vi "PFI-28000-28144-Demo_Main.vi"() -> ()   [LabVIEW 2017]
uses:
  PFI-28000-28144-Demo-State.ctl
  PFI-28000-28144-Demo-State Data.ctl
  28144 Card/PFI-28000-Card-28144.lvclass
  C:/wc/07143 Precision Filters 28000 Support/Driver/source/Card/PFI-28000-Card.lvclass
  28144 Channel/PFI-28000-Chan-28144.lvclass
  C:/wc/07143 Precision Filters 28000 Support/Driver/source/Bridge Channel/PFI-28000-Chan-Bridge.lvclass
  Card/PFI-28000-Card.lvclass
  Channel/PFI-28000-Channel.lvclass
  System/PFI-28000-System.lvclass
panel:
  in  "Type":enum16{"Low Pass Only", "Band Pass"}(ring)
  out "Auto Bal Status":string[](array[string])
  in  "Stop":bool
  in  "Auto Balance":bool[](array[boolean])
  out "Loop Resistance":dbl[](array[numeric])
  out "Excitation Current":dbl[](array[numeric])
  out "Identity":string
  out "Hostname":string
  in  "Gain":dbl[](array[numeric])
  in  "LP Filter Cutoff":dbl[](array[numeric])
  in  "Port":u16=28000
  in  "Address":string="169.254.1.221"
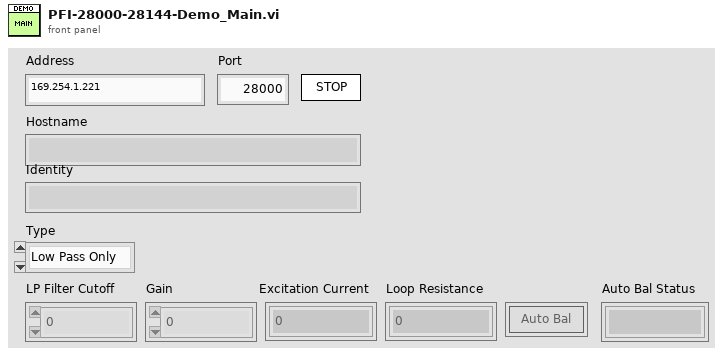
[diagram p1: front panel]
types:
  T1 = typedef "PFI-28000-28144-Demo-State Data.ctl" = cluster{"Card":refnum<class "PFI-28000-Card-28144.lvclass">, "Channels":refnum<class "PFI-28000-Chan-28144.lvclass">[]}
  T2 = typedef "PFI-28000-28144-Demo-State.ctl" = enum16{"InitDevice", "InitGUI", "HandleEvent"}
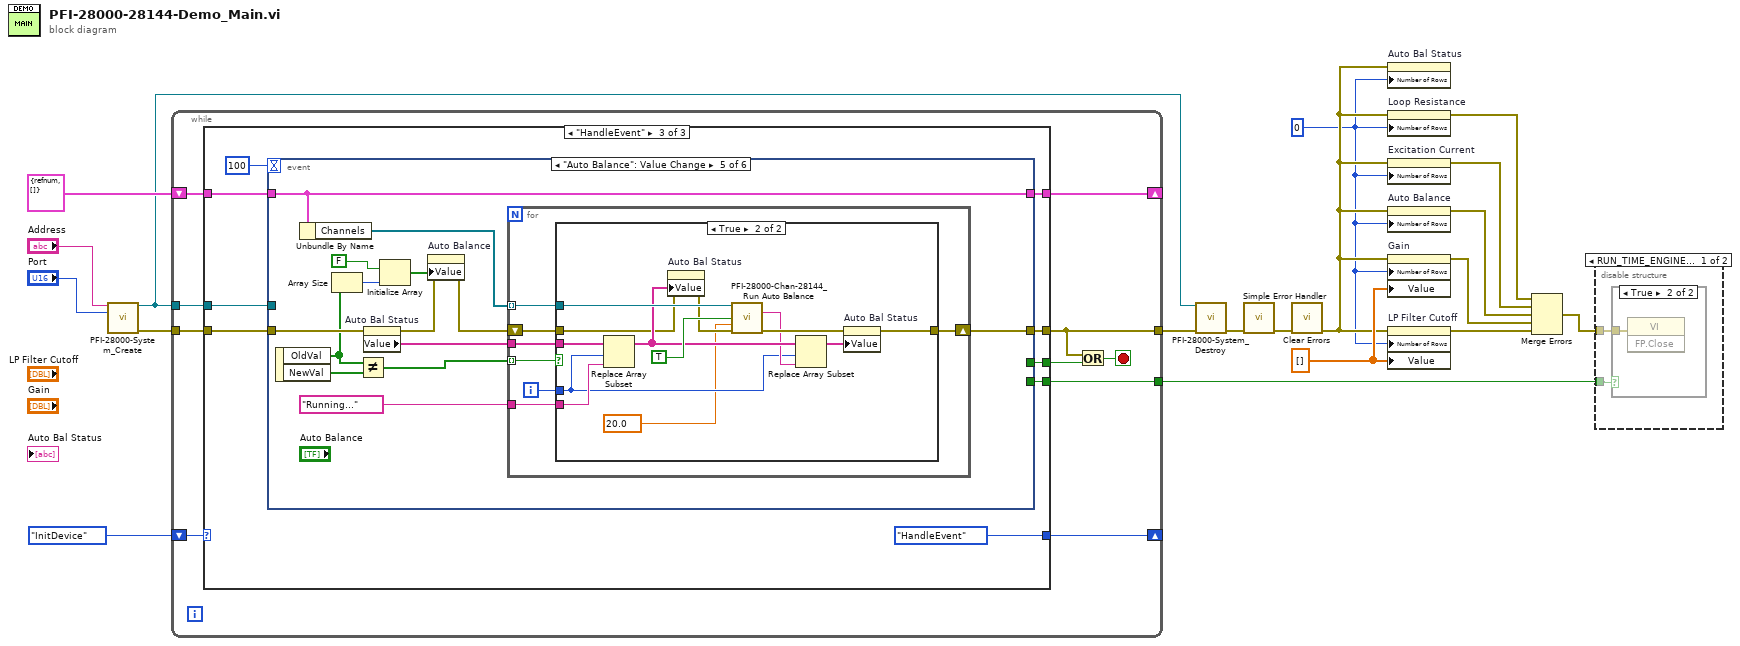
[diagram p0: block diagram]
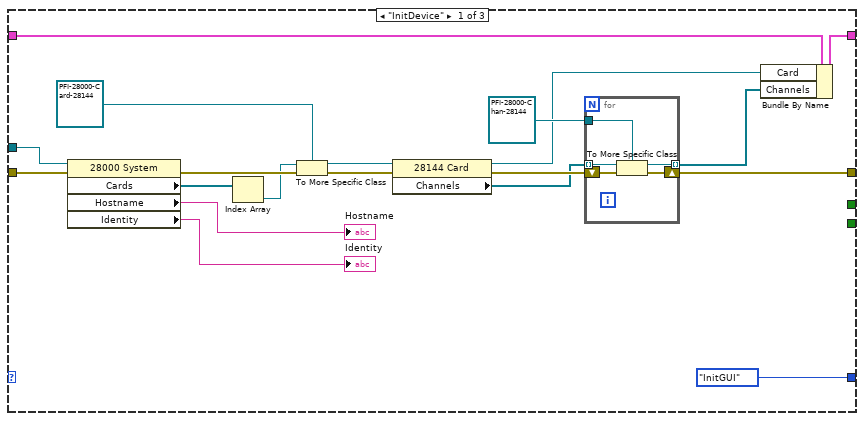
[diagram p4: hidden frame]
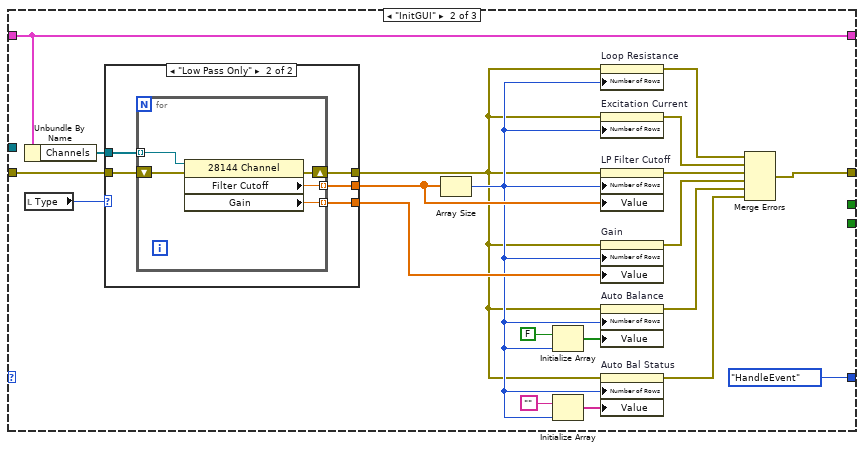
[diagram p5: hidden frame]
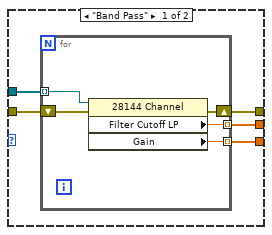
[diagram p6: hidden frame]
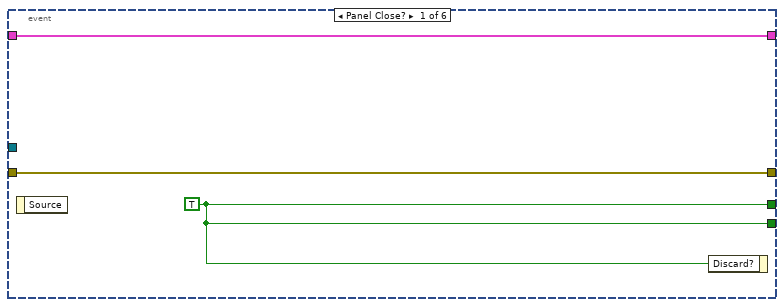
[diagram p7: hidden frame]
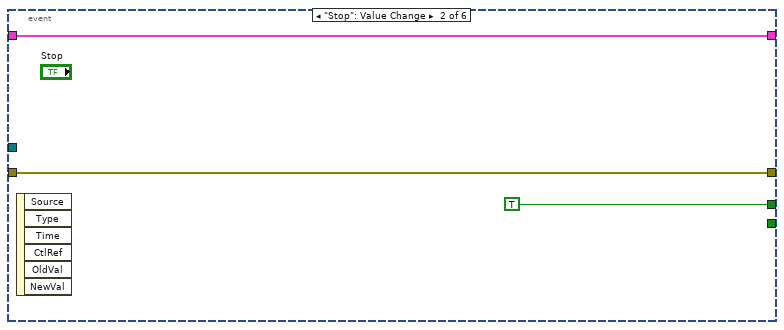
[diagram p8: hidden frame]
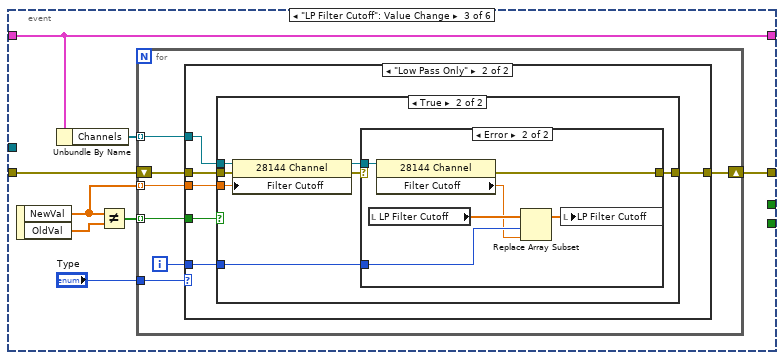
[diagram p9: hidden frame]
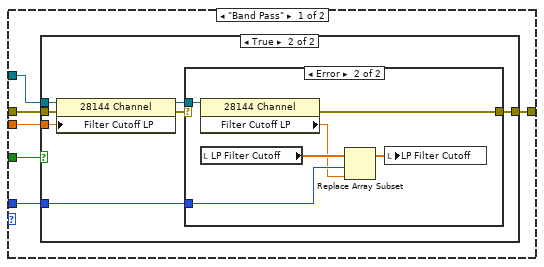
[diagram p10: hidden frame]
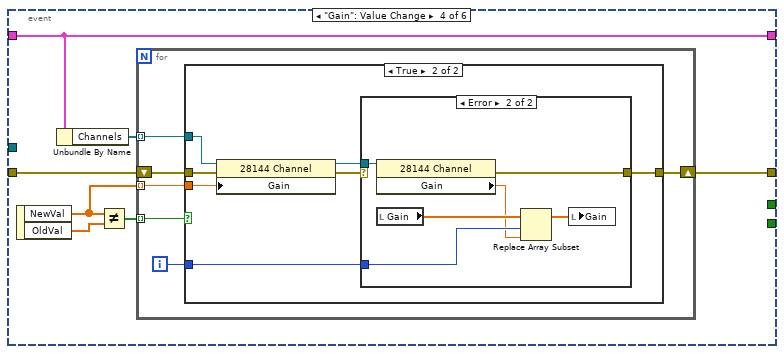
[diagram p15: hidden frame]
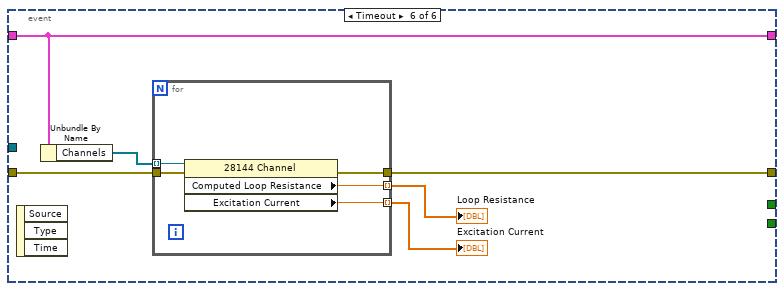
[diagram p19: hidden frame]
diagram:
  w10 = dbl[] [] ("Filter Cutoff")
  w2 = u32 0 ("Number of Rows")
  n1 = call "PFI-28000-System_Create.vi"("Address"="Address", "Port"="Port") -> ("PFI-28000-System out"=w13:refnum<class "PFI-28000-System.lvclass">, "error out"=w17:errorcluster)  [unwired: 12 in]
  n2 = while {
    tunnel: w17 -> [w29]
    tunnel: w13 -> [w27]
    shift-right: [w26] -> _
    shift-left: PFI-28000-28144-Demo-State."InitDevice" -> [w28]
    shift-right: [w24] -> _
    shift-left: T1 {"Card"=refnum, "Channels"=[]} ("Data") -> [w25]
    tunnel: [w23] -> w14
    tunnel: [w20] -> w1
    stop <- w22 stop-if-true
    n3 = case shown="\"HandleEvent\"" w28 {
      tunnel: w27 -> [w48 _ w102]
      tunnel: w29 -> [w47 w72 w101]
      tunnel: [PFI-28000-28144-Demo-State."InitGUI" PFI-28000-28144-Demo-State."HandleEvent" PFI-28000-28144-Demo-State."HandleEvent"] -> w26
      tunnel: [w37 w62 w98] -> w23
      tunnel: w25 -> [w36 w73 w97]
      tunnel: [w35 w73 w96] -> w24
      tunnel: [_ _ w99] -> w21
      tunnel: [_ _ w94] -> w20
      frame "InitDevice" {
        n4 = property class="28000 System"(reference=w48, error in=w47) -> (error out=w45:errorcluster, "Cards"=w46:refnum<class "PFI-28000-Card.lvclass">[], "Hostname"=→"Hostname":string, "Identity"=→"Identity":string)  [unwired: 1 out]
        n5 = Index Array(array=w46) -> (element=w44:refnum<class "PFI-28000-Card.lvclass">)  [unwired: 1 in]
        n6 = To More Specific Class(target class=refnum<class "PFI-28000-Card-28144.lvclass"> refnum ("PFI-28000-Card-28144.lvclass"), reference=w44, error in=w45) -> (specific class reference=w42:refnum<class "PFI-28000-Card-28144.lvclass">, error out=w41:errorcluster)
        n7 = property class="28144 Card"(reference=w42, error in=w41) -> (reference out=w33:refnum<class "PFI-28000-Card-28144.lvclass">, error out=w40:errorcluster, "Channels"=w34:refnum<class "PFI-28000-Channel.lvclass">[])
        n8 = for {
          shift-right: [w50] -> w37
          shift-left: w40 -> [w53]
          tunnel: w34 -> [w52] mode=indexing
          tunnel: refnum<class "PFI-28000-Chan-28144.lvclass"> refnum ("PFI-28000-Chan-28144.lvclass") -> [w51]
          tunnel: [w49] -> w32 mode=indexing
          n9 = To More Specific Class(target class=w51, reference=w52, error in=w53) -> (specific class reference=w49:refnum<class "PFI-28000-Chan-28144.lvclass">, error out=w50:errorcluster)
        }
        n10 = Bundle By Name(cluster=w36, "Card"=w33, "Channels"=w32) -> (w35:T1)
      }
      frame "InitGUI" {
        n11 = Unbundle By Name(w73) -> ("Channels"=w71:refnum<class "PFI-28000-Chan-28144.lvclass">[])
        n12 = local read "Type"() -> (w54:enum16{"Low Pass Only", "Band Pass"})
        n13 = case shown="\"Low Pass Only\"" w54 {
          tunnel: w72 -> [w78 w88]
          tunnel: w71 -> [w77 w87]
          tunnel: [w76 w86] -> w69
          tunnel: [w75 w85] -> w68
          tunnel: [w74 w84] -> w56
          frame "Band Pass" {
            n14 = for {
              shift-right: [w81] -> w74
              shift-left: w78 -> [w83]
              tunnel: w77 -> [w82] mode=indexing
              tunnel: [w80] -> w76 mode=indexing
              tunnel: [w79] -> w75 mode=indexing
              n15 = property class="28144 Channel"(reference=w82, error in=w83) -> (error out=w81:errorcluster, "Filter Cutoff LP"=w80:dbl, "Gain"=w79:dbl)  [unwired: 1 out]
            }
          }
          frame "Low Pass Only" {
            n16 = for {
              shift-right: [w91] -> w84
              shift-left: w88 -> [w93]
              tunnel: w87 -> [w92] mode=indexing
              tunnel: [w90] -> w86 mode=indexing
              tunnel: [w89] -> w85 mode=indexing
              n17 = property class="28144 Channel"(reference=w92, error in=w93) -> (error out=w91:errorcluster, "Filter Cutoff"=w90:dbl, "Gain"=w89:dbl)  [unwired: 1 out]
            }
          }
        }
        n18 = Array Size(array=w69) -> (size(s)=w57:i32)
        n19 = Initialize Array(FALSE, w57) -> (w60:bool[])
        n20 = Initialize Array("", w57) -> (w58:string[])
        n21 = property on="Loop Resistance" class="Arr (strict)"(error in=w56, "Number of Rows"=w57) -> (error out=w63:errorcluster)  [unwired: 1 in, 1 out]
        n22 = property on="Excitation Current" class="Arr (strict)"(error in=w56, "Number of Rows"=w57) -> (error out=w64:errorcluster)  [unwired: 1 in, 1 out]
        n23 = property on="LP Filter Cutoff" class="Arr (strict)"(error in=w56, "Number of Rows"=w57, "Value"=w69) -> (error out=w67:errorcluster)  [unwired: 1 in, 1 out]
        n24 = property on="Gain" class="Arr (strict)"(error in=w56, "Number of Rows"=w57, "Value"=w68) -> (error out=w66:errorcluster)  [unwired: 1 in, 1 out]
        n25 = property on="Auto Balance" class="Arr"(error in=w56, "Number of Rows"=w57, "Value"=w60) -> (error out=w65:errorcluster)  [unwired: 1 in, 1 out]
        n26 = property on="Auto Bal Status" class="Arr (strict)"(error in=w56, "Number of Rows"=w57, "Value"=w58) -> (error out=w55:errorcluster)  [unwired: 1 in, 1 out]
        n27 = Merge Errors(w63, w64, w67, w66, w65, w55) -> (w62:errorcluster)
      }
      frame "HandleEvent" {
        n28 = event shown="[4] \"Auto Balance\": Value Change" {
          selector: _ -> [_ _ _ _ _ _]
          dyn-events: _ -> [_ _ _ _ _ _]
          timeout: 100 -> [_ _ _ _ _ _]
          tunnel: w102 -> [_ _ _ _ _ _]
          tunnel: w101 -> [w105 w108 w115 w171 w202 w233]
          tunnel: [w103 TRUE _ _ _ _] -> w99
          tunnel: [w105 w108 w112 w168 w204 w231] -> w98
          tunnel: [w104 w107 w116 w172 w206 w234] -> w96
          tunnel: w97 -> [w104 w107 w116 w172 w206 w234]
          tunnel: [w103 _ _ _ _ _] -> w94
          event Panel Close? {
            w103 = TRUE
            n29 = event-data() -> ()  [unwired: 1 in, 1 out]
            n30 = event-data("Discard?"=w103) -> ()  [unwired: 1 in, 1 out]
          }
          event "Stop": Value Change {
            n31 = event-data() -> ()  [unwired: 1 in, 6 out]
          }
          event "LP Filter Cutoff": Value Change {
            n32 = event-data() -> ("NewVal"=w111:dbl[], "OldVal"=w110:dbl[])  [unwired: 1 in]
            n33 = Unbundle By Name(w116) -> ("Channels"=w114:refnum<class "PFI-28000-Chan-28144.lvclass">[])
            n34 = Not Equal?(x=w111, y=w110) -> (x != y?=w113:bool[])
            n35 = for {
              shift-right: [w121] -> w112
              shift-left: w115 -> [w123]
              tunnel: w114 -> [w122] mode=indexing
              tunnel: w113 -> [w120] mode=indexing
              tunnel: w111 -> [w119] mode=indexing
              tunnel: "Type" -> [w117]
              i -> [w118]
              n36 = case shown="\"Low Pass Only\"" w117 {
                tunnel: w123 -> [w129 w150]
                tunnel: w122 -> [w128 w149]
                tunnel: [w126 w147] -> w121
                tunnel: w119 -> [w127 w148]
                tunnel: w118 -> [w125 w146]
                tunnel: w120 -> [w124 w145]
                frame "Band Pass" {
                  n37 = case shown="True" w124 {
                    tunnel: w129 -> [w130 w137]
                    tunnel: w128 -> [_ w136]
                    tunnel: w127 -> [_ w135]
                    tunnel: [w130 w133] -> w126
                    tunnel: w125 -> [_ w132]
                    frame False {
                    }
                    frame True {
                      n38 = property class="28144 Channel"(reference=w136, error in=w137, "Filter Cutoff LP"=w135) -> (reference out=w131:refnum<class "PFI-28000-Chan-28144.lvclass">, error out=w134:errorcluster)
                      n39 = case shown="Error" w134 {
                        selector: w134 -> [w138 _]
                        tunnel: [w138 w139] -> w133
                        tunnel: w132 -> [_ w144]
                        tunnel: w131 -> [_ w141]
                        frame No Error {
                        }
                        frame Error {
                          n40 = property class="28144 Channel"(reference=w141) -> (error out=w139:errorcluster, "Filter Cutoff LP"=w140:dbl)  [unwired: 1 in, 1 out]
                          n41 = local read "LP Filter Cutoff"() -> (w143:dbl[])
                          n42 = Replace Array Subset(array=w143, new element=w140, index=w144) -> (w142:dbl[])
                          n43 = local write "LP Filter Cutoff"(w142) -> ()
                        }
                      }
                    }
                  }
                }
                frame "Low Pass Only" {
                  n44 = case shown="True" w145 {
                    tunnel: w150 -> [w151 w158]
                    tunnel: w149 -> [_ w157]
                    tunnel: w148 -> [_ w156]
                    tunnel: [w151 w154] -> w147
                    tunnel: w146 -> [_ w153]
                    frame False {
                    }
                    frame True {
                      n45 = property class="28144 Channel"(reference=w157, error in=w158, "Filter Cutoff"=w156) -> (reference out=w152:refnum<class "PFI-28000-Chan-28144.lvclass">, error out=w155:errorcluster)
                      n46 = case shown="Error" w155 {
                        selector: w155 -> [w159 _]
                        tunnel: [w159 w160] -> w154
                        tunnel: w153 -> [_ w165]
                        tunnel: w152 -> [_ w162]
                        frame No Error {
                        }
                        frame Error {
                          n47 = local read "LP Filter Cutoff"() -> (w164:dbl[])
                          n48 = property class="28144 Channel"(reference=w162) -> (error out=w160:errorcluster, "Filter Cutoff"=w161:dbl)  [unwired: 1 in, 1 out]
                          n49 = Replace Array Subset(array=w164, new element=w161, index=w165) -> (w163:dbl[])
                          n50 = local write "LP Filter Cutoff"(w163) -> ()
                        }
                      }
                    }
                  }
                }
              }
            }
          }
          event "Gain": Value Change {
            n51 = event-data() -> ("NewVal"=w167:dbl[], "OldVal"=w166:dbl[])  [unwired: 1 in]
            n52 = Unbundle By Name(w172) -> ("Channels"=w170:refnum<class "PFI-28000-Chan-28144.lvclass">[])
            n53 = Not Equal?(x=w167, y=w166) -> (x != y?=w169:bool[])
            n54 = for {
              shift-right: [w176] -> w168
              shift-left: w171 -> [w178]
              tunnel: w170 -> [w177] mode=indexing
              tunnel: w169 -> [w175] mode=indexing
              tunnel: w167 -> [w174] mode=indexing
              i -> [w173]
              n55 = case shown="True" w175 {
                tunnel: w178 -> [w179 w186]
                tunnel: w177 -> [_ w185]
                tunnel: [w179 w182] -> w176
                tunnel: w174 -> [_ w184]
                tunnel: w173 -> [_ w181]
                frame False {
                }
                frame True {
                  n56 = property class="28144 Channel"(reference=w185, error in=w186, "Gain"=w184) -> (reference out=w180:refnum<class "PFI-28000-Chan-28144.lvclass">, error out=w183:errorcluster)
                  n57 = case shown="Error" w183 {
                    selector: w183 -> [w187 _]
                    tunnel: [w187 w189] -> w182
                    tunnel: w181 -> [_ w193]
                    tunnel: w180 -> [_ w190]
                    frame No Error {
                    }
                    frame Error {
                      n58 = property class="28144 Channel"(reference=w190) -> (error out=w189:errorcluster, "Gain"=w188:dbl)  [unwired: 1 in, 1 out]
                      n59 = local read "Gain"() -> (w192:dbl[])
                      n60 = Replace Array Subset(array=w192, new element=w188, index=w193) -> (w191:dbl[])
                      n61 = local write "Gain"(w191) -> ()
                    }
                  }
                }
              }
            }
          }
          event "Auto Balance": Value Change {
            n62 = event-data() -> ("OldVal"=w197:bool[], "NewVal"=w207:bool[])  [unwired: 1 in]
            n63 = Unbundle By Name(w206) -> ("Channels"=w205:refnum<class "PFI-28000-Chan-28144.lvclass">[])
            n64 = Array Size(array=w197) -> (size(s)=w198:i32)
            n65 = Not Equal?(x=w197, y=w207) -> (x != y?=w203:bool[])
            n66 = property on="Auto Bal Status" class="Arr (strict)"(error in=w202) -> (error out=w195:errorcluster, "Value"=w201:string[])  [unwired: 1 in, 1 out]
            n67 = Initialize Array(FALSE, w198) -> (w199:bool[])
            n68 = property on="Auto Balance" class="Arr"(error in=w195, "Value"=w199) -> (error out=w194:errorcluster)  [unwired: 1 in, 1 out]
            n69 = for {
              shift-right: [w212] -> w204
              shift-left: w194 -> [w213]
              tunnel: w205 -> [w214] mode=indexing
              tunnel: w203 -> [w211] mode=indexing
              tunnel: w201 -> [w210]
              tunnel: "Running..." ("empty string") -> [w208]
              i -> [w209]
              n70 = case shown="True" w211 {
                tunnel: w214 -> [_ w228]
                tunnel: w213 -> [w215 w220]
                tunnel: [w215 w223] -> w212
                tunnel: w210 -> [_ w226]
                tunnel: w209 -> [_ w218]
                tunnel: w208 -> [_ w221]
                frame False {
                }
                frame True {
                  n71 = Replace Array Subset(array=w226, new element=w221, index=w218) -> (w222:string[])
                  n72 = property on="Auto Bal Status" class="Arr (strict)"(error in=w220, "Value"=w222) -> (error out=w225:errorcluster)  [unwired: 1 in, 1 out]
                  n73 = call-dynamic "PFI-28000-Chan-28144_Run Auto Balance.vi"("PFI-28000-Chan-28144 in"=w228, "Wait For Done"=TRUE, "Timeout"=20.0 ("Auto Bal Timeout"), "error in (no error)"=w225) -> ("Result"=w219:string, "error out"=w224:errorcluster)  [unwired: 9 in, 1 out]
                  n74 = Replace Array Subset(array=w222, new element=w219, index=w218) -> (w217:string[])
                  n75 = property on="Auto Bal Status" class="Arr (strict)"(error in=w224, "Value"=w217) -> (error out=w223:errorcluster)  [unwired: 1 in, 1 out]
                }
              }
            }
          }
          event Timeout {
            n76 = event-data() -> ()  [unwired: 1 in, 3 out]
            n77 = Unbundle By Name(w234) -> ("Channels"=w232:refnum<class "PFI-28000-Chan-28144.lvclass">[])
            n78 = for {
              tunnel: w232 -> [w239] mode=indexing
              tunnel: [w237] -> w229 mode=indexing
              tunnel: [w236] -> w230 mode=indexing
              tunnel: w233 -> [w238]
              tunnel: [w235] -> w231
              n79 = property class="28144 Channel"(reference=w239, error in=w238) -> (error out=w235:errorcluster, "Computed Loop Resistance"=w237:dbl, "Excitation Current"=w236:dbl)  [unwired: 1 out]
            }
            "Excitation Current" <- w230
            "Loop Resistance" <- w229
          }
        }
      }
    }
    n80 = Or(x=w23, y=w21) -> (x .or. y?=w22:bool)
  }
  n81 = call-dynamic "PFI-28000-System_Destroy.vi"("PFI-28000-System in"=w13, "error in (no error)"=w14) -> ("error out"=w12:errorcluster)  [unwired: 13 in]
  n82 = call <vilib>:"Simple Error Handler.vi"("error in (no error)"=w12) -> ("error out"=w11:errorcluster)  [unwired: 4 in, 4 out]
  n83 = call <vilib>:"Clear Errors.vi"("error in (no error)"=w11) -> ("error out"=w3:errorcluster)  [unwired: 5 in, 1 out]
  n84 = property on="Auto Bal Status" class="Arr (strict)"(error in=w3, "Number of Rows"=w2) -> ()  [unwired: 1 in, 2 out]
  n85 = property on="Loop Resistance" class="Arr (strict)"(error in=w3, "Number of Rows"=w2) -> (error out=w5:errorcluster)  [unwired: 1 in, 1 out]
  n86 = property on="Excitation Current" class="Arr (strict)"(error in=w3, "Number of Rows"=w2) -> (error out=w6:errorcluster)  [unwired: 1 in, 1 out]
  n87 = property on="Auto Balance" class="Arr"(error in=w3, "Number of Rows"=w2) -> (error out=w7:errorcluster)  [unwired: 1 in, 1 out]
  n88 = property on="Gain" class="Arr (strict)"(error in=w3, "Number of Rows"=w2, "Value"=w10) -> (error out=w8:errorcluster)  [unwired: 1 in, 1 out]
  n89 = property on="LP Filter Cutoff" class="Arr (strict)"(error in=w3, "Number of Rows"=w2, "Value"=w10) -> (error out=w9:errorcluster)  [unwired: 1 in, 1 out]
  n90 = Merge Errors(w5, w6, w7, w8, w9) -> (w4:errorcluster)
  n91 = disable-structure shown="RUN_TIME_ENGINE==True" {
    disable-tunnel: w4 -> [w241 _]
    disable-tunnel: w1 -> [w240 _]
    frame condition #0 {
      n92 = case shown="True" w240 {
        tunnel: w241 -> [_ w242]
        frame False {
        }
        frame True {
          n93 = invoke class="VI" method="FP.Close"(error in=w242) -> ()  [unwired: 2 in, 3 out]
        }
      }
    }
    frame condition #1 (active) {
    }
  }
